vi "ShooterFullPower.vi"(2 "Button":bool, 3 "RearMotorPowerIn":dbl, 4 "FrontMotorPowerIn":dbl) -> (0 "FrontMotorPowerOut":dbl, 1 "RearMotorPowerOut":dbl)   [LabVIEW 2016]
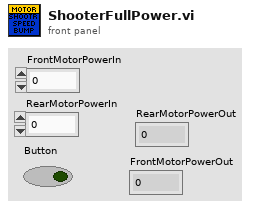
[diagram p1: front panel]
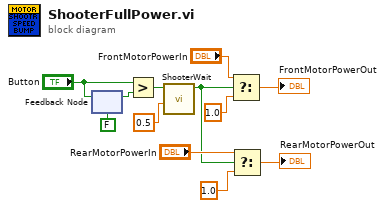
[diagram p0: block diagram]
diagram:
  n1 = feedback-in #1("Button") -> ()
  n2 = feedback #1(FALSE ("Button")) -> (w11:bool)
  n3 = Greater?(x="Button", y=w11) -> (0:w12:bool)
  n4 = call "ShooterWait.vi"("Target Time (s)"=0.5, "First Time?"=w12) -> ("Completed"=w2:bool)  [unwired: 8 in, 1 out]
  n5 = Select(t="FrontMotorPowerIn", s=w2, f=1.0 ("t")) -> (s? t:f=→"FrontMotorPowerOut":dbl)
  n6 = Select(t="RearMotorPowerIn", s=w2, f=1.0 ("t")) -> (s? t:f=→"RearMotorPowerOut":dbl)
